vi "Stop.vi"   [LabVIEW 2021]
uses:
  <vilib>/event_ctls.llb/usereventprio.ctl
types:
  T1 = typedef "usereventprio.ctl" = enum32{"high priority", "normal priority"}
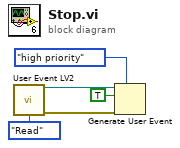
[diagram p0: block diagram]
diagram:
  n1 = call "User Event LV2.vi"("LV2 operations"=enum16{"Read", "Write"}."Read") -> ("Stop event out"=w4:refnum<user-event>, "error out"=w2:errorcluster)  [unwired: 13 in]
  n2 = Generate User Event(priority (normal)=usereventprio."high priority", user event=w4, event data cluster=TRUE ("event data"), error in=w2) -> ()  [unwired: 2 out]
